vi "CSM - Resolve Node Module.vi"(10 "Node Name":string) -> (2 "CSM Module Name":string)   [LabVIEW 2017, in "Communicable State Machine.lvlib"]
uses:
  Communicable State Machine.lvlib
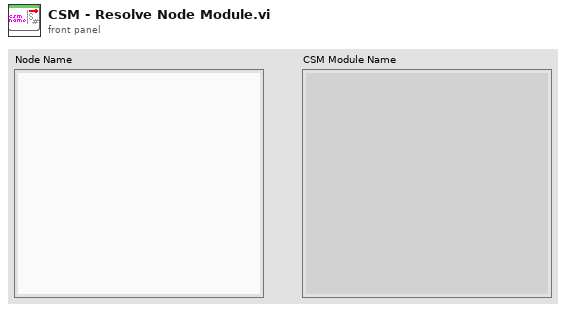
[diagram p1: front panel]
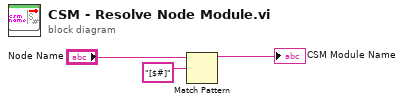
[diagram p0: block diagram]
diagram:
  n1 = Match Pattern(string="Node Name", regular expression="[$#]") -> (before substring=→"CSM Module Name":string)  [unwired: 1 in, 3 out]
